vi "dynamic mapping.vi"(8 "error in":errorcluster, 10 "channels available":refnum<class "TBM channel.lvclass">[](array[class]), 11 "asynchronous execution module configuration In":refnum<class "asynchronous execution module configuration.lvclass">) -> (0 "error out":errorcluster, 2 "reservations":T1[](array[typedef]), 3 "asynchronous execution module configuration Out":refnum<class "asynchronous execution module configuration.lvclass">)   [LabVIEW 2013, in "asynchronous execution module configuration.lvclass"]
doc: "Provides an interface for dynamically mapping data at runtime instead of static mapping. For example, a component may which to log all data in a given execution system to disk. In this case, it would register to read data from all groups defined as inputs to the system. Calling code is responsible for providing this data to the requesting component. There is no way to \"undo\" reservations within a component without directly manipulating the component's data."
uses:
  asynchronous execution module configuration.lvclass
  <vilib>/NI/Tag Bus Module Framework/module configuration/channel reservation.ctl
  <vilib>/NI/Tag Bus Module Framework/channel/TBM channel.lvclass
  asynchronous execution module configuration.lvclass/asynchronous execution module configuration.ctl
  <vilib>/NI/Tag Bus Module Framework/module configuration/TBM module configuration.lvclass
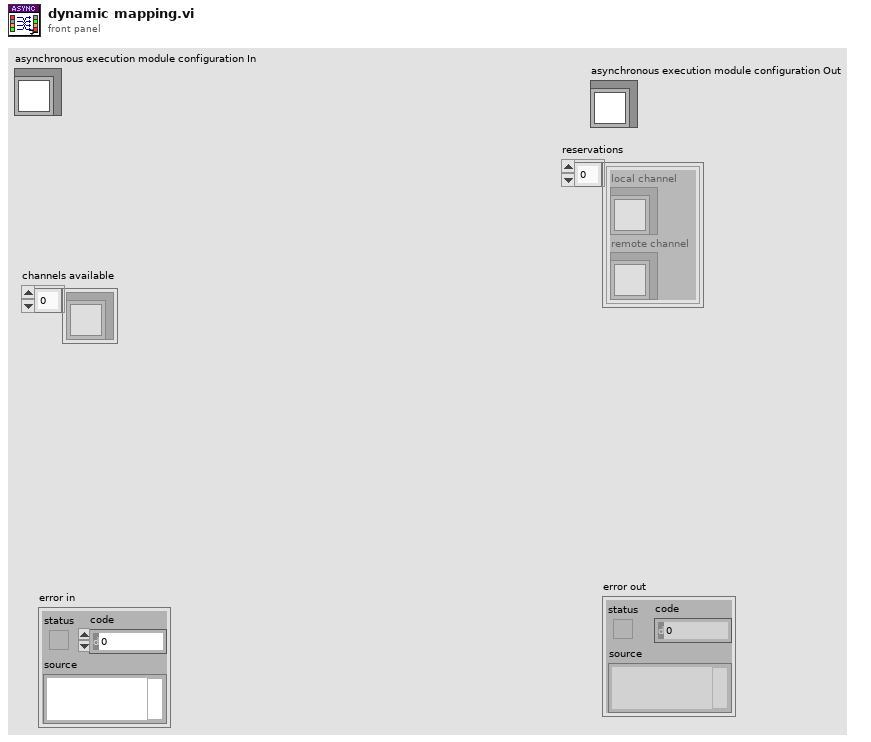
[diagram p1: front panel]
types:
  T1 = typedef "TBM module configuration.lvclass/channel reservation.ctl" = cluster{"local channel":refnum<class "TBM channel.lvclass">, "remote channel":refnum<class "TBM channel.lvclass">}
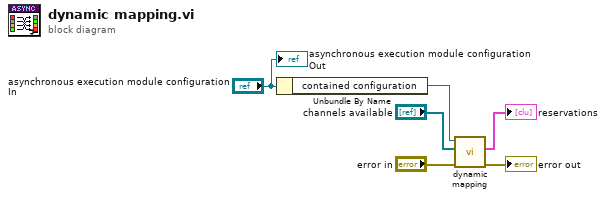
[diagram p0: block diagram]
diagram:
  n1 = Unbundle By Name("asynchronous execution module configuration In") -> ("contained configuration"=w5:refnum<class "TBM module configuration.lvclass">)
  n2 = call-dynamic "dynamic mapping.vi"("error in"="error in", "channels available"="channels available", "module configuration in"=w5) -> ("error out"=→"error out":errorcluster, "reservations"=→"reservations":T1[])  [unwired: 6 in, 1 out]
  "asynchronous execution module configuration Out" <- "asynchronous execution module configuration In"
